vi "cam_process.vi"(0 "image in":T2) -> (6 "# of green targets":i32, 8 "# of red targets":i32, 9 "# of Blue targets":i32, 10 "# of Yellow targets":i32, 12 "# of Orange targets":i32, 14 "image with hud":T2, 15 "green":cluster{"x-point":dbl, "y-point":dbl}[](array[cluster]), 16 "red":cluster{"x-point":dbl, "y-point":dbl}[](array[cluster]), 17 "yellow":cluster{"x-point":dbl, "y-point":dbl}[](array[cluster]), 18 "blue":cluster{"x-point":dbl, "y-point":dbl}[](array[cluster]), 19 "orange":cluster{"x-point":dbl, "y-point":dbl}[](array[cluster]))   [LabVIEW 2018]
uses:
  <vilib>/vision/Image Controls.llb/IMAQ Image.ctl
panel:
  in  "Tab Control":T1(tab)
  out "XY Graph 2":cluster{dbl[], dbl[]}[](graph)
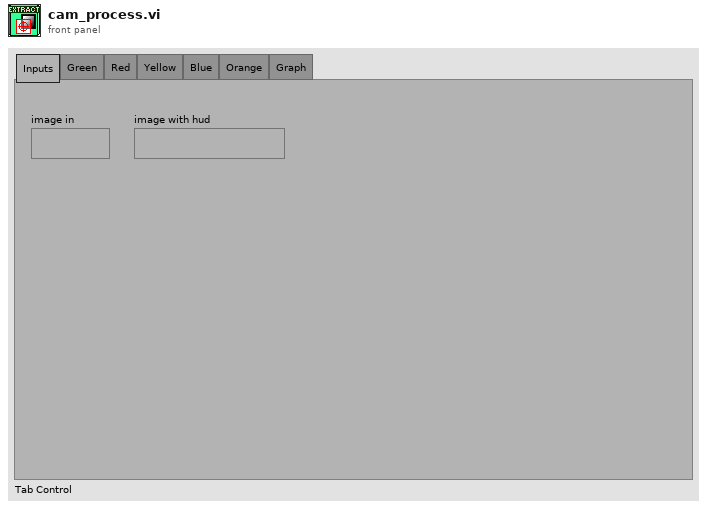
[diagram p1: front panel]
types:
  T1 = enum32{"Inputs", "Green", "Red", "Yellow", "Blue", "Orange", "Graph"}
  T2 = typedef "IMAQ Image.ctl" = refnum<image>
  T3 = typedef "Image Type" = u32
  T4 = cluster{"Left":i32, "Top":i32, "Right":i32, "Bottom":i32}
  T5 = cluster{"Particle Measurements (Pixels) (green targets)[0]":dbl, "Particle Measurements (Pixels) (green targets)[1]":dbl, "Particle Measurements (Pixels) (green targets)[2]":dbl, "Particle Measurements (Pixels) (green targets)[3]":dbl, "Particle Measurements (Pixels) (green targets)[4]":dbl, "Particle Measurements (Pixels) (green targets)[5]":dbl, "Particle Measurements (Pixels) (green targets)[6]":dbl, "Particle Measurements (Pixels) (green targets)[7]":dbl, "Particle Measurements (Pixels) (green targets)[8]":dbl}
  T6 = cluster{"Particle Measurements (Pixels) (red targets)[0]":dbl, "Particle Measurements (Pixels) (red targets)[1]":dbl, "Particle Measurements (Pixels) (red targets)[2]":dbl, "Particle Measurements (Pixels) (red targets)[3]":dbl, "Particle Measurements (Pixels) (red targets)[4]":dbl, "Particle Measurements (Pixels) (red targets)[5]":dbl, "Particle Measurements (Pixels) (red targets)[6]":dbl, "Particle Measurements (Pixels) (red targets)[7]":dbl, "Particle Measurements (Pixels) (red targets)[8]":dbl}
  T7 = cluster{"Particle Measurements (Pixels) (Yellow targets)[0]":dbl, "Particle Measurements (Pixels) (Yellow targets)[1]":dbl, "Particle Measurements (Pixels) (Yellow targets)[2]":dbl, "Particle Measurements (Pixels) (Yellow targets)[3]":dbl, "Particle Measurements (Pixels) (Yellow targets)[4]":dbl, "Particle Measurements (Pixels) (Yellow targets)[5]":dbl, "Particle Measurements (Pixels) (Yellow targets)[6]":dbl, "Particle Measurements (Pixels) (Yellow targets)[7]":dbl, "Particle Measurements (Pixels) (Yellow targets)[8]":dbl}
  T8 = cluster{"Particle Measurements (Pixels) (Blue targets)[0]":dbl, "Particle Measurements (Pixels) (Blue targets)[1]":dbl, "Particle Measurements (Pixels) (Blue targets)[2]":dbl, "Particle Measurements (Pixels) (Blue targets)[3]":dbl, "Particle Measurements (Pixels) (Blue targets)[4]":dbl, "Particle Measurements (Pixels) (Blue targets)[5]":dbl, "Particle Measurements (Pixels) (Blue targets)[6]":dbl, "Particle Measurements (Pixels) (Blue targets)[7]":dbl, "Particle Measurements (Pixels) (Blue targets)[8]":dbl}
  T9 = cluster{"Particle Measurements (Pixels) (Orange targets)[0]":dbl, "Particle Measurements (Pixels) (Orange targets)[1]":dbl, "Particle Measurements (Pixels) (Orange targets)[2]":dbl, "Particle Measurements (Pixels) (Orange targets)[3]":dbl, "Particle Measurements (Pixels) (Orange targets)[4]":dbl, "Particle Measurements (Pixels) (Orange targets)[5]":dbl, "Particle Measurements (Pixels) (Orange targets)[6]":dbl, "Particle Measurements (Pixels) (Orange targets)[7]":dbl, "Particle Measurements (Pixels) (Orange targets)[8]":dbl}
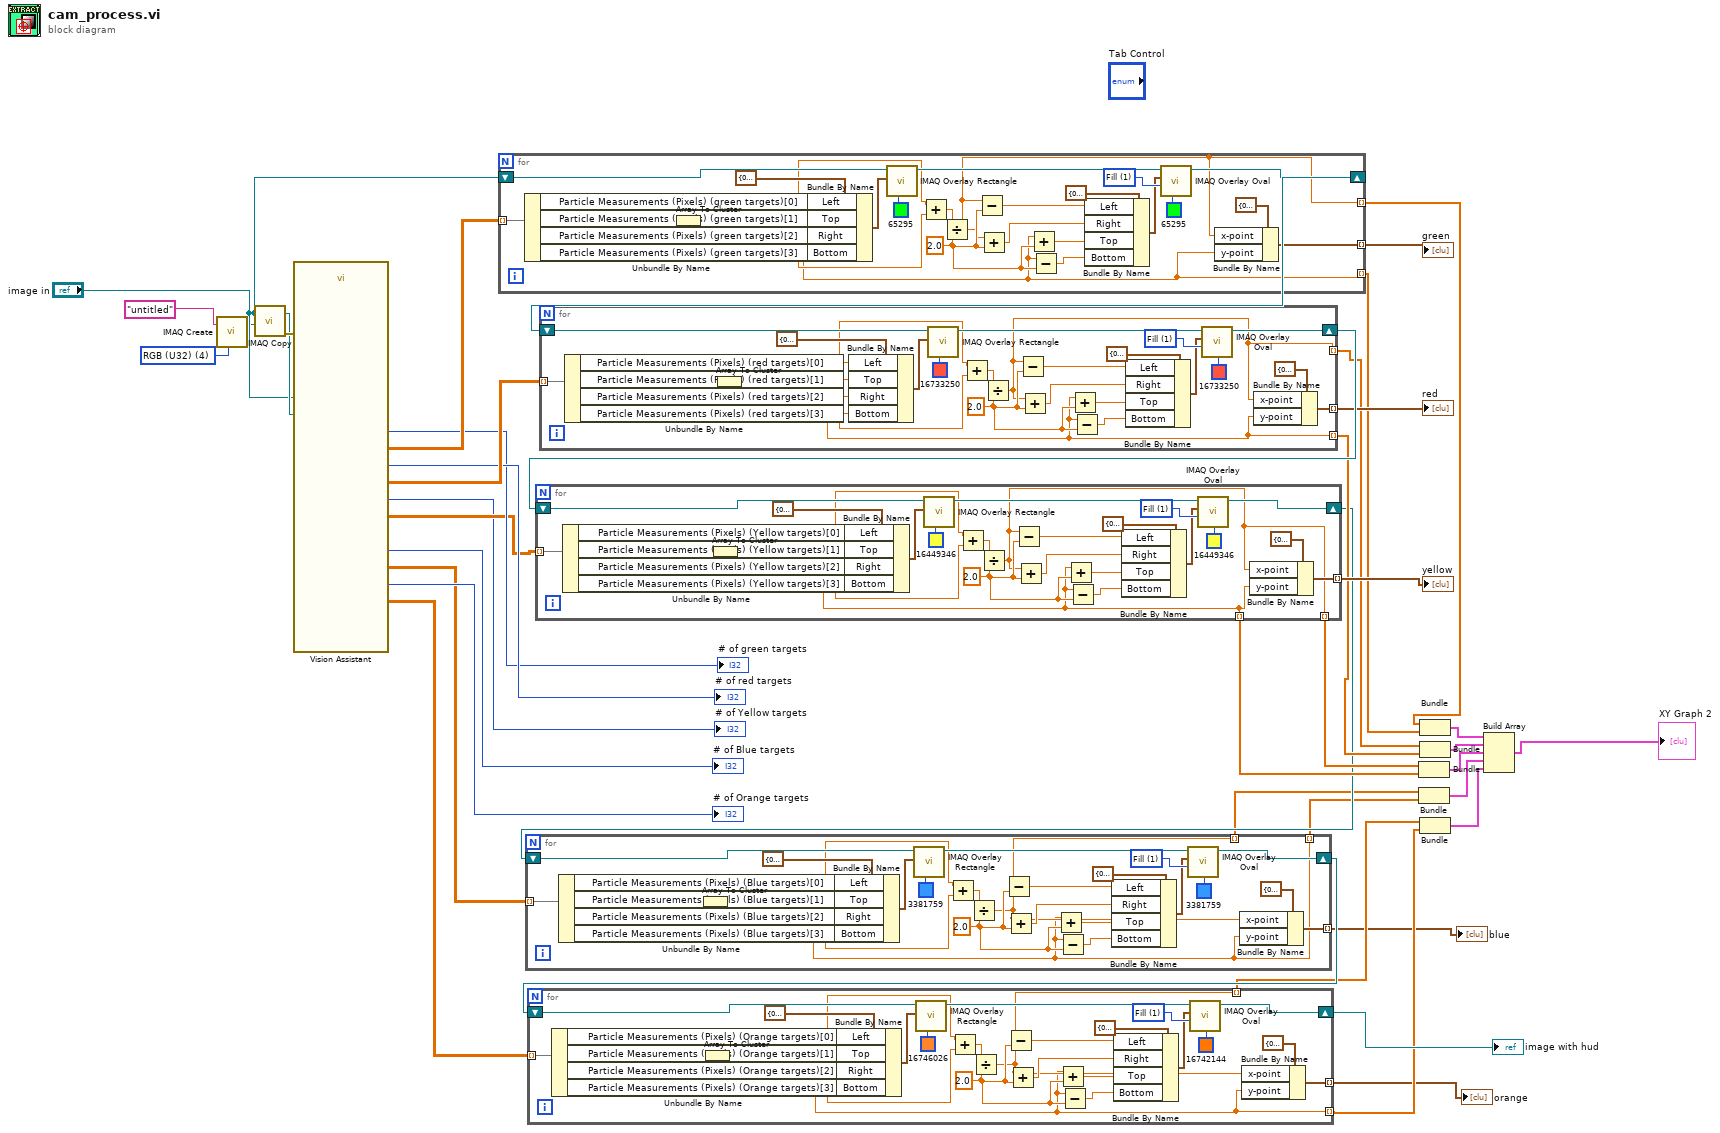
[diagram p0: block diagram]
diagram:
  w38 = T3 4 items=["Grayscale (U8)", "Grayscale (I16)", "Grayscale (SGL)", "Complex (CSG)", "RGB (U32)", "HSL (U32)", "RGB (U64)", "Grayscale (U16)"] ("Image Type")
  n1 = call "IMAQ Create"("Image Name"="untitled", "Image Type"=w38) -> ("New Image"=w29:T2)  [unwired: 3 in, 1 out]
  n2 = call "IMAQ Copy"("Image Dst"=w29, "Image Src"="image in") -> ("error out"=w39:errorcluster, "Image Dst Out"=w31:T2)  [unwired: 4 in]
  n3 = call "Vision Assistant"("Image In"="image in", "Image Dst"=w31, "error in"=w39) -> ("Particle Measurements (Pixels) (Orange targets)"=w12:dbl[][], "Number of Particles (Orange targets)"=→"# of Orange targets":i32, "Particle Measurements (Pixels) (Blue targets)"=w13:dbl[][], "Number of Particles (Blue targets)"=→"# of Blue targets":i32, "Number of Particles (green targets)"=→"# of green targets":i32, "Particle Measurements (Pixels) (green targets)"=w40:dbl[][], "Number of Particles (red targets)"=→"# of red targets":i32, "Particle Measurements (Pixels) (red targets)"=w42:dbl[][], "Number of Particles (Yellow targets)"=→"# of Yellow targets":i32, "Particle Measurements (Pixels) (Yellow targets)"=w34:dbl[][])  [unwired: 13 in, 2 out]
  n4 = for {
    tunnel: w40 -> [w64] mode=indexing
    shift-right: [w45] -> w41
    shift-left: "image in" -> [w67]
    tunnel: [w46] -> w26 mode=indexing
    tunnel: [w44] -> w25 mode=indexing
    tunnel: [w43] -> w24 mode=indexing
    w51 = 2.0 ("y")
    w59 = u32 1 items=["Frame", "Fill"] ("Drawing Mode (Frame)")
    n5 = Array To Cluster(array=w64) -> (cluster=w63:T5)
    n6 = Unbundle By Name(w63) -> ("Particle Measurements (Pixels) (green targets)[0]"=w55:dbl, "Particle Measurements (Pixels) (green targets)[1]"=w62:dbl, "Particle Measurements (Pixels) (green targets)[2]"=w54:dbl, "Particle Measurements (Pixels) (green targets)[3]"=w43:dbl)
    n7 = Bundle By Name(cluster=T4 {"Left"=0, "Top"=0, "Right"=0, "Bottom"=0} ("Rectangle"), "Left"=w55, "Top"=w62, "Right"=w54, "Bottom"=w43) -> (w65:T4)
    n8 = call "IMAQ Overlay Rectangle"("Color"=u32 65295, "Rectangle"=w65, "Image"=w67) -> ("Image Out"=w60:T2)  [unwired: 7 in, 1 out]
    n9 = Add(x=w55, y=w54) -> (x+y=w56:dbl)
    n10 = Divide(x=w56, y=w51) -> (x/y=w44:dbl)
    n11 = Subtract(x=w44, y=w51) -> (x-y=w53:dbl)
    n12 = Add(x=w44, y=w51) -> (x+y=w52:dbl)
    n13 = Add(x=w43, y=w51) -> (x+y=w50:dbl)
    n14 = Subtract(x=w43, y=w51) -> (x-y=w49:dbl)
    n15 = Bundle By Name(cluster=T4 {"Left"=0, "Top"=0, "Right"=0, "Bottom"=0} ("Bounding Rectangle"), "Left"=w53, "Right"=w52, "Top"=w50, "Bottom"=w49) -> (w58:T4)
    n16 = call "IMAQ Overlay Oval"("Color"=u32 65295, "Drawing Mode (Frame)"=w59, "Bounding Rectangle"=w58, "Image"=w60) -> ("Image Out"=w45:T2)  [unwired: 6 in, 1 out]
    n17 = Bundle By Name(cluster=cluster{"x-point":dbl, "y-point":dbl} {"x-point"=0.0, "y-point"=0.0} ("input cluster"), "x-point"=w44, "y-point"=w43) -> (w46:cluster{"x-point":dbl, "y-point":dbl})
  }
  "green" <- w26
  n18 = for {
    tunnel: w42 -> [w89] mode=indexing
    shift-right: [w70] -> w32
    shift-left: w41 -> [w92]
    tunnel: [w71] -> w28 mode=indexing
    tunnel: [w69] -> w21 mode=indexing
    tunnel: [w68] -> w20 mode=indexing
    w77 = 2.0 ("y")
    w85 = u32 1 items=["Frame", "Fill"] ("Drawing Mode (Frame)")
    n19 = Array To Cluster(array=w89) -> (cluster=w88:T6)
    n20 = Unbundle By Name(w88) -> ("Particle Measurements (Pixels) (red targets)[0]"=w81:dbl, "Particle Measurements (Pixels) (red targets)[1]"=w87:dbl, "Particle Measurements (Pixels) (red targets)[2]"=w80:dbl, "Particle Measurements (Pixels) (red targets)[3]"=w68:dbl)
    n21 = Bundle By Name(cluster=T4 {"Left"=0, "Top"=0, "Right"=0, "Bottom"=0} ("Rectangle"), "Left"=w81, "Top"=w87, "Right"=w80, "Bottom"=w68) -> (w90:T4)
    n22 = call "IMAQ Overlay Rectangle"("Color"=u32 16733250, "Rectangle"=w90, "Image"=w92) -> ("Image Out"=w86:T2)  [unwired: 7 in, 1 out]
    n23 = Add(x=w81, y=w80) -> (x+y=w82:dbl)
    n24 = Divide(x=w82, y=w77) -> (x/y=w69:dbl)
    n25 = Subtract(x=w69, y=w77) -> (x-y=w79:dbl)
    n26 = Add(x=w69, y=w77) -> (x+y=w78:dbl)
    n27 = Add(x=w68, y=w77) -> (x+y=w76:dbl)
    n28 = Subtract(x=w68, y=w77) -> (x-y=w75:dbl)
    n29 = Bundle By Name(cluster=T4 {"Left"=0, "Top"=0, "Right"=0, "Bottom"=0} ("Bounding Rectangle"), "Left"=w79, "Right"=w78, "Top"=w76, "Bottom"=w75) -> (w84:T4)
    n30 = call "IMAQ Overlay Oval"("Color"=u32 16733250, "Drawing Mode (Frame)"=w85, "Bounding Rectangle"=w84, "Image"=w86) -> ("Image Out"=w70:T2)  [unwired: 6 in, 1 out]
    n31 = Bundle By Name(cluster=cluster{"x-point":dbl, "y-point":dbl} {"x-point"=0.0, "y-point"=0.0} ("input cluster"), "x-point"=w69, "y-point"=w68) -> (w71:cluster{"x-point":dbl, "y-point":dbl})
  }
  "red" <- w28
  n32 = for {
    tunnel: w34 -> [w114] mode=indexing
    shift-right: [w110] -> w9
    shift-left: w32 -> [w117]
    tunnel: [w95] -> w27 mode=indexing
    tunnel: [w94] -> w17 mode=indexing
    tunnel: [w93] -> w16 mode=indexing
    w101 = 2.0 ("y")
    w109 = u32 1 items=["Frame", "Fill"] ("Drawing Mode (Frame)")
    n33 = Array To Cluster(array=w114) -> (cluster=w113:T7)
    n34 = Unbundle By Name(w113) -> ("Particle Measurements (Pixels) (Yellow targets)[0]"=w105:dbl, "Particle Measurements (Pixels) (Yellow targets)[1]"=w112:dbl, "Particle Measurements (Pixels) (Yellow targets)[2]"=w104:dbl, "Particle Measurements (Pixels) (Yellow targets)[3]"=w93:dbl)
    n35 = Bundle By Name(cluster=T4 {"Left"=0, "Top"=0, "Right"=0, "Bottom"=0} ("Rectangle"), "Left"=w105, "Top"=w112, "Right"=w104, "Bottom"=w93) -> (w115:T4)
    n36 = call "IMAQ Overlay Rectangle"("Color"=u32 16449346, "Rectangle"=w115, "Image"=w117) -> ("Image Out"=w111:T2)  [unwired: 7 in, 1 out]
    n37 = Add(x=w105, y=w104) -> (x+y=w106:dbl)
    n38 = Divide(x=w106, y=w101) -> (x/y=w94:dbl)
    n39 = Subtract(x=w94, y=w101) -> (x-y=w103:dbl)
    n40 = Add(x=w94, y=w101) -> (x+y=w102:dbl)
    n41 = Add(x=w93, y=w101) -> (x+y=w100:dbl)
    n42 = Subtract(x=w93, y=w101) -> (x-y=w99:dbl)
    n43 = Bundle By Name(cluster=T4 {"Left"=0, "Top"=0, "Right"=0, "Bottom"=0} ("Bounding Rectangle"), "Left"=w103, "Right"=w102, "Top"=w100, "Bottom"=w99) -> (w108:T4)
    n44 = call "IMAQ Overlay Oval"("Color"=u32 16449346, "Drawing Mode (Frame)"=w109, "Bounding Rectangle"=w108, "Image"=w111) -> ("Image Out"=w110:T2)  [unwired: 6 in, 1 out]
    n45 = Bundle By Name(cluster=cluster{"x-point":dbl, "y-point":dbl} {"x-point"=0.0, "y-point"=0.0} ("input cluster"), "x-point"=w94, "y-point"=w93) -> (w95:cluster{"x-point":dbl, "y-point":dbl})
  }
  "yellow" <- w27
  n46 = for {
    tunnel: w13 -> [w139] mode=indexing
    shift-right: [w135] -> w10
    shift-left: w9 -> [w142]
    tunnel: [w120] -> w2 mode=indexing
    tunnel: [w119] -> w8 mode=indexing
    tunnel: [w118] -> w7 mode=indexing
    w126 = 2.0 ("y")
    w134 = u32 1 items=["Frame", "Fill"] ("Drawing Mode (Frame)")
    n47 = Array To Cluster(array=w139) -> (cluster=w138:T8)
    n48 = Unbundle By Name(w138) -> ("Particle Measurements (Pixels) (Blue targets)[0]"=w130:dbl, "Particle Measurements (Pixels) (Blue targets)[1]"=w137:dbl, "Particle Measurements (Pixels) (Blue targets)[2]"=w129:dbl, "Particle Measurements (Pixels) (Blue targets)[3]"=w118:dbl)
    n49 = Bundle By Name(cluster=T4 {"Left"=0, "Top"=0, "Right"=0, "Bottom"=0} ("Rectangle"), "Left"=w130, "Top"=w137, "Right"=w129, "Bottom"=w118) -> (w140:T4)
    n50 = call "IMAQ Overlay Rectangle"("Color"=u32 3381759, "Rectangle"=w140, "Image"=w142) -> ("Image Out"=w136:T2)  [unwired: 7 in, 1 out]
    n51 = Add(x=w130, y=w129) -> (x+y=w131:dbl)
    n52 = Divide(x=w131, y=w126) -> (x/y=w119:dbl)
    n53 = Subtract(x=w119, y=w126) -> (x-y=w128:dbl)
    n54 = Add(x=w119, y=w126) -> (x+y=w127:dbl)
    n55 = Add(x=w118, y=w126) -> (x+y=w125:dbl)
    n56 = Subtract(x=w118, y=w126) -> (x-y=w124:dbl)
    n57 = Bundle By Name(cluster=T4 {"Left"=0, "Top"=0, "Right"=0, "Bottom"=0} ("Bounding Rectangle"), "Left"=w128, "Right"=w127, "Top"=w125, "Bottom"=w124) -> (w133:T4)
    n58 = call "IMAQ Overlay Oval"("Color"=u32 3381759, "Drawing Mode (Frame)"=w134, "Bounding Rectangle"=w133, "Image"=w136) -> ("Image Out"=w135:T2)  [unwired: 6 in, 1 out]
    n59 = Bundle By Name(cluster=cluster{"x-point":dbl, "y-point":dbl} {"x-point"=0.0, "y-point"=0.0} ("input cluster"), "x-point"=w119, "y-point"=w118) -> (w120:cluster{"x-point":dbl, "y-point":dbl})
  }
  "blue" <- w2
  n60 = for {
    tunnel: w12 -> [w164] mode=indexing
    shift-right: [w160] -> w11
    shift-left: w10 -> [w167]
    tunnel: [w145] -> w1 mode=indexing
    tunnel: [w144] -> w6 mode=indexing
    tunnel: [w143] -> w5 mode=indexing
    w151 = 2.0 ("y")
    w159 = u32 1 items=["Frame", "Fill"] ("Drawing Mode (Frame)")
    n61 = Array To Cluster(array=w164) -> (cluster=w163:T9)
    n62 = Unbundle By Name(w163) -> ("Particle Measurements (Pixels) (Orange targets)[0]"=w155:dbl, "Particle Measurements (Pixels) (Orange targets)[1]"=w162:dbl, "Particle Measurements (Pixels) (Orange targets)[2]"=w154:dbl, "Particle Measurements (Pixels) (Orange targets)[3]"=w143:dbl)
    n63 = Bundle By Name(cluster=T4 {"Left"=0, "Top"=0, "Right"=0, "Bottom"=0} ("Rectangle"), "Left"=w155, "Top"=w162, "Right"=w154, "Bottom"=w143) -> (w165:T4)
    n64 = call "IMAQ Overlay Rectangle"("Color"=u32 16746026, "Rectangle"=w165, "Image"=w167) -> ("Image Out"=w161:T2)  [unwired: 7 in, 1 out]
    n65 = Add(x=w155, y=w154) -> (x+y=w156:dbl)
    n66 = Divide(x=w156, y=w151) -> (x/y=w144:dbl)
    n67 = Subtract(x=w144, y=w151) -> (x-y=w153:dbl)
    n68 = Add(x=w144, y=w151) -> (x+y=w152:dbl)
    n69 = Add(x=w143, y=w151) -> (x+y=w150:dbl)
    n70 = Subtract(x=w143, y=w151) -> (x-y=w149:dbl)
    n71 = Bundle By Name(cluster=T4 {"Left"=0, "Top"=0, "Right"=0, "Bottom"=0} ("Bounding Rectangle"), "Left"=w153, "Right"=w152, "Top"=w150, "Bottom"=w149) -> (w158:T4)
    n72 = call "IMAQ Overlay Oval"("Color"=u32 16742144, "Drawing Mode (Frame)"=w159, "Bounding Rectangle"=w158, "Image"=w161) -> ("Image Out"=w160:T2)  [unwired: 6 in, 1 out]
    n73 = Bundle By Name(cluster=cluster{"x-point":dbl, "y-point":dbl} {"x-point"=0.0, "y-point"=0.0} ("input cluster"), "x-point"=w144, "y-point"=w143) -> (w145:cluster{"x-point":dbl, "y-point":dbl})
  }
  "image with hud" <- w11
  "orange" <- w1
  n74 = Bundle(w17, w16) -> (w18:cluster{dbl[], dbl[]})  [unwired: 1 in]
  n75 = Bundle(w8, w7) -> (w4:cluster{dbl[], dbl[]})  [unwired: 1 in]
  n76 = Bundle(w25, w24) -> (w23:cluster{dbl[], dbl[]})  [unwired: 1 in]
  n77 = Bundle(w21, w20) -> (w19:cluster{dbl[], dbl[]})  [unwired: 1 in]
  n78 = Bundle(w6, w5) -> (w3:cluster{dbl[], dbl[]})  [unwired: 1 in]
  n79 = Build Array(w23, w19, w18, w4, w3) -> (→"XY Graph 2":cluster{dbl[], dbl[]}[])
